vi "Convert Unix Time To LabVIEW time.vi"(2 "String":dbl) -> (6 "date/time string":string)   [LabVIEW 2019]
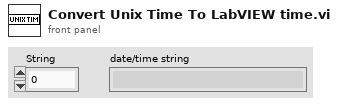
[diagram p1: front panel]
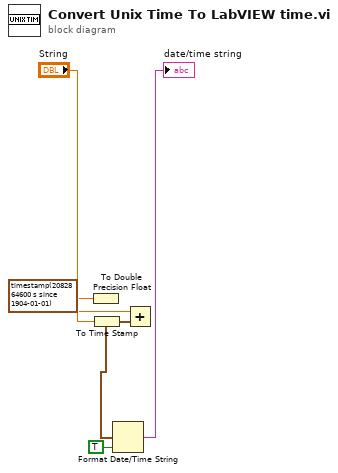
[diagram p0: block diagram]
diagram:
  n1 = To Double Precision Float(number=timestamp(2082864600 s since 1904-01-01) ("time stamp 2")) -> (double precision float=w4:dbl)
  n2 = To Time Stamp(1:"String") -> (0:w2:timestamp)
  n3 = Add(x=w4, y=w2) -> (x+y=w3:timestamp)
  n4 = Format Date/Time String(seconds (now)=w3, UTC format=TRUE) -> (date/time string=→"date/time string":string)  [unwired: 1 in]
